vi "High Speed Stream With Replicate.vi"() -> ()   [LabVIEW 2023]
doc: "This VI demonstrates an advanced use of the High Speed Pipe, showing how a single channel can be replicated to feed data to multiple receivers."
uses:
  <vilib>/ChannelSupport/Channel Abort Instructions.ctl
  <extravilib>/ChannelInstances/High Speed Stream-i32/Abort Signal/Abort Signal.lvclass/Abort Signal.ctl
  <extravilib>/ChannelInstances/High Speed Stream-i32/_Read For Replicate.vi
  <extravilib>/ChannelInstances/High Speed Stream-i32/Instantiate.vi
  <extravilib>/ChannelInstances/High Speed Stream-i32/)Channel.vi
  <extravilib>/ChannelInstances/High Speed Stream-i32/Abort Signal/Init Signal.vi
  <extravilib>/ChannelInstances/High Speed Stream-i32.lvlib
  <extravilib>/ChannelInstances/High Speed Stream-i32/Abort Signal/Abort Signal.lvclass
panel:
  in  "Independent Abort?":bool
  in  "Delay 1":u32=50
  in  "Delay 2":u32=100
  in  "Stop Consumer 2":bool
  out "Data Consumed 2":i32(graph)
  in  "Consumer Stop Value 2":i32=-1
  in  "Consumer Stop Value":i32=-1
  in  "Emergency Stop Producer":bool
  out "Data Consumed":i32(graph)
  out "Data Produced":i32(graph)
  in  "Stop Consumer":bool
  in  "Stop Producer":bool
  # "Overview: This VI assumes you have already looked at the other VI in this project: High Speed Stream.vi.\nThis VI shows the use of the Replicate function. A single High Speed Stream goes in; two such Streams come out. The content of the original pipe is duplicated so that both of the replicas get their own copy of the data. The replicas start off consuming the data at different rates. This example lets you see the effects of different rates of consumption on the system overall. Notice that with a bounded buffer, the consumer loops will tend to synchronize because data can only be replicated at the rate of the slowest consumer loop.\nInstructions:\n1. Configure the two Delay values for the two consumer loops. Select whether the loops have independent abort or not.\n2. Run the VI. Press the Normal Stop Producer button to see the producer stop; the consumers both continue until they each catch up.\n3. Run the VI again. The Emergency Stop Producer button will halt all the consumers as quickly as possible.\n3. Run the VI again. Any of the other stop conditions depend upon the \"Independent Abort?\" setting. If it is false then the two replicas share an abort signal: aborting one for any reason will abort the other. If it is true then one replica can stop but the producer will continue producing data for the other one."
  # "Set These Before Running VI"
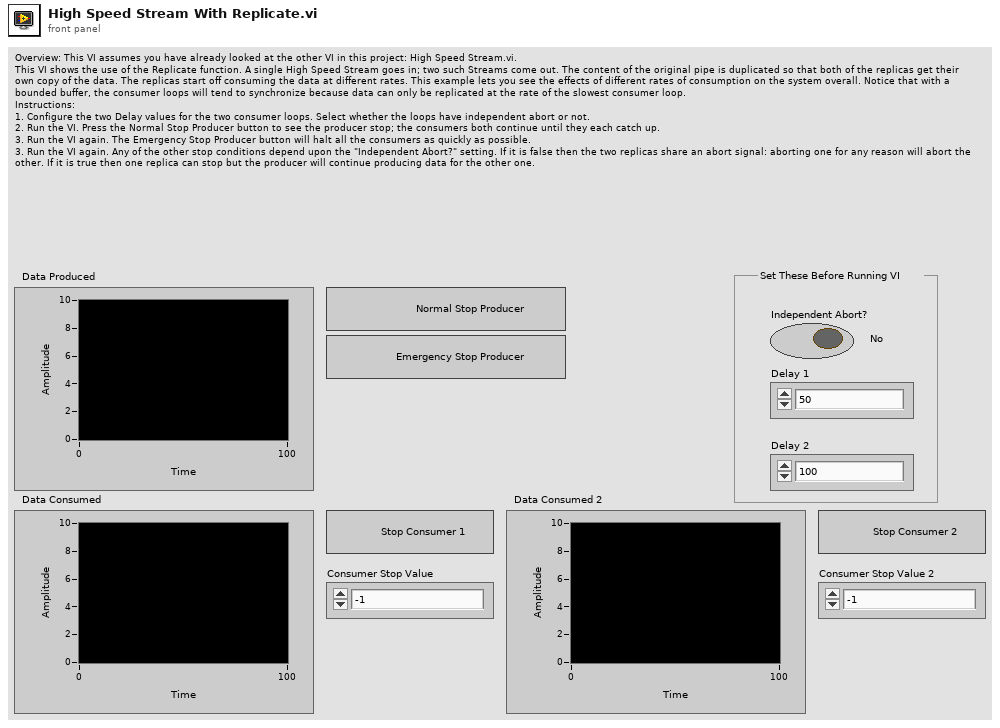
[diagram p1: front panel]
types:
  T1 = typedef "Channel Abort Instructions.ctl" = enum16{"No abort", "Abort now", "Abort if timeout"}
  T2 = typedef "High Speed Stream-i32.lvlib/)Channel.ctl" = refnum<queue>
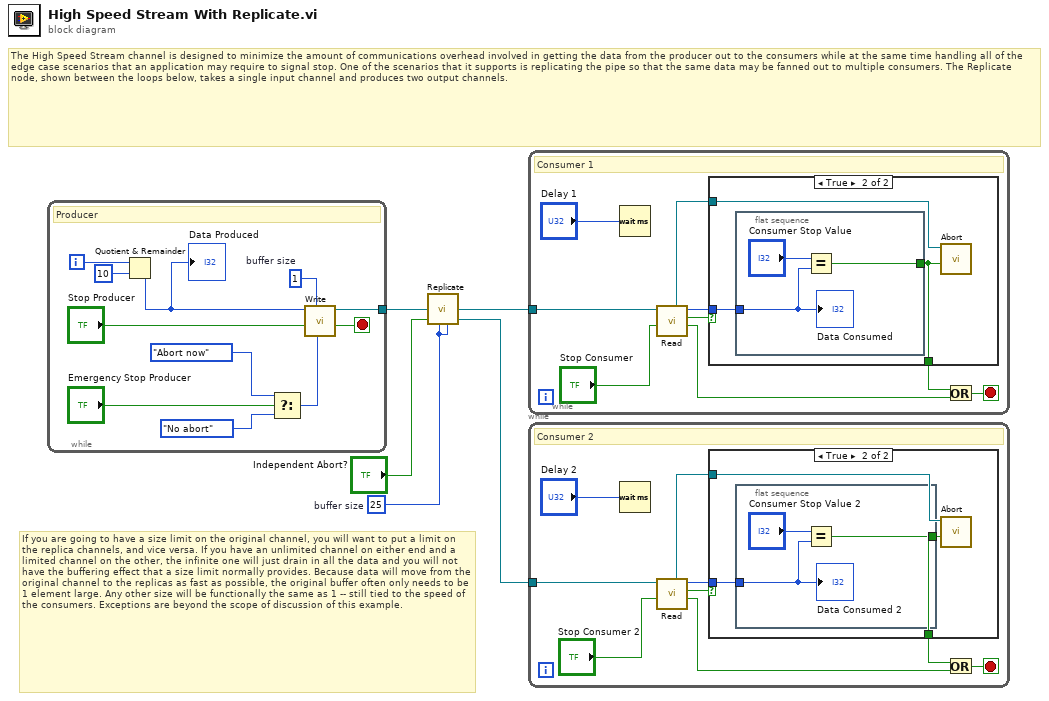
[diagram p0: block diagram]
diagram:
  w4 = 25  # buffer size
  # "If you are going to have a size limit on the original channel, you will want to put a limit on the replica channels, and vice versa. If you have an unlimited channel on either end and a limited channel on the other, the infinite one will just drain in all the data and you will not have the buffering effect that a size limit normally provides. Because data will move from the original channel to the replicas as fast as possible, the original buffer often only needs to be 1 element large. Any other size will be functionally the same as 1 -- still tied to the speed of the consumers. Exceptions are beyond the scope of discussion of this example."
  # "The High Speed Stream channel is designed to minimize the amount of communications overhead involved in getting the data from the producer out to the consumers while at the same time handling all of the edge case scenarios that an application may require to signal stop. One of the scenarios that it supports is replicating the pipe so that the same data may be fanned out to multiple consumers. The Replicate node, shown between the loops below, takes a single input channel and produces two output channels."
  n1 = while {
    tunnel: [w9] -> w5
    i -> [w12]
    stop <- w8 stop-if-true
    w10 = 1  # buffer size
    # "Producer"
    n2 = Quotient & Remainder(x=w12, y=10) -> (x-y*floor(x/y)=w11:i32)  [unwired: 1 out]
    "Data Produced" <- w11
    n3 = Select(t=Channel_Abort_Instructions."Abort now" ("abort instructions (no abort)"), s="Emergency Stop Producer", f=Channel_Abort_Instructions."No abort" ("abort instructions (no abort)")) -> (s? t:f=w7:T1)
    n4 = call <extravilib>:"Write.vi"("abort status (no abort)"=w7, "size (unlimited)"=w10, "last element? (F)"="Stop Producer", "element"=w11) -> ("done?"=w8:bool, "channel"=w9:T2)  [unwired: 5 in, 1 out]
  }
  n5 = call <extravilib>:"Replicate.vi"("high speed stream"=w5, "independent aborts? (F)"="Independent Abort?", "copy 1 size (unlimited)"=w4, "copy 2 size (unlimited)"=w4) -> ("high speed stream copy 1"=w1:T2, "high speed stream copy 2"=w2:T2)  [unwired: 4 in]
  n6 = while {
    tunnel: w1 -> [w22]
    stop <- w25 stop-if-true
    # "Consumer 1"
    n7 = Wait (ms)(milliseconds to wait="Delay 1") -> ()  [unwired: 1 out]
    n8 = call <extravilib>:"Read.vi"("abort before read? (F)"="Stop Consumer", "channel"=w22) -> ("done?"=w19:bool, "element valid?"=w17:bool, "element"=w18:i32, "abort signal"=w21:refnum<class "Abort Signal.lvclass">)  [unwired: 5 in, 1 out]
    n9 = case shown="True" w17 {
      tunnel: w21 -> [_ w27]
      tunnel: w18 -> [_ w28]
      tunnel: [_ w26] -> w24
      frame False {
      }
      frame True {
        n10 = flat-sequence {
          tunnel: w28 -> [w30]
          tunnel: [w29] -> w26
          frame #0 {
            n11 = Equal?(x="Consumer Stop Value", y=w30) -> (x = y?=w29:bool)
            "Data Consumed" <- w30
          }
        }
        n12 = call <extravilib>:"Abort.vi"("abort? (T)"=w26, "abort signal"=w27) -> ()  [unwired: 9 in, 1 out]
      }
    }
    n13 = Or(x=w24, y=w19) -> (x .or. y?=w25:bool)
  }
  n14 = while {
    tunnel: w2 -> [w37]
    stop <- w40 stop-if-true
    # "Consumer 2"
    n15 = Wait (ms)(milliseconds to wait="Delay 2") -> ()  [unwired: 1 out]
    n16 = call <extravilib>:"Read.vi"("abort before read? (F)"="Stop Consumer 2", "channel"=w37) -> ("done?"=w34:bool, "element valid?"=w32:bool, "element"=w35:i32, "abort signal"=w36:refnum<class "Abort Signal.lvclass">)  [unwired: 5 in, 1 out]
    n17 = case shown="True" w32 {
      tunnel: w36 -> [_ w41]
      tunnel: w35 -> [_ w43]
      tunnel: [_ w42] -> w39
      frame False {
      }
      frame True {
        n18 = flat-sequence {
          tunnel: w43 -> [w45]
          tunnel: [w44] -> w42
          frame #0 {
            n19 = Equal?(x="Consumer Stop Value 2", y=w45) -> (x = y?=w44:bool)
            "Data Consumed 2" <- w45
          }
        }
        n20 = call <extravilib>:"Abort.vi"("abort? (T)"=w42, "abort signal"=w41) -> ()  [unwired: 9 in, 1 out]
      }
    }
    n21 = Or(x=w39, y=w34) -> (x .or. y?=w40:bool)
  }
